vi "Get Data.vi"(8 "error in (no error)":errorcluster, 11 "Red Pitaya Digitizer in":refnum<class "Red Pitaya Digitizer.lvclass">) -> (0 "error out":errorcluster, 3 "Red Pitaya Digitizer out":refnum<class "Red Pitaya Digitizer.lvclass">)   [LabVIEW 2015, in "Red Pitaya Digitizer.lvclass"]
uses:
  Red Pitaya Digitizer.lvclass
  Red Pitaya Digitizer.lvclass/Red Pitaya Digitizer.ctl
  Read RP Instrument.lvclass.vi
  NHMFL_Core/Libraries/Red Pitaya/RP Core/RP Instrument/RP Instrument.lvclass
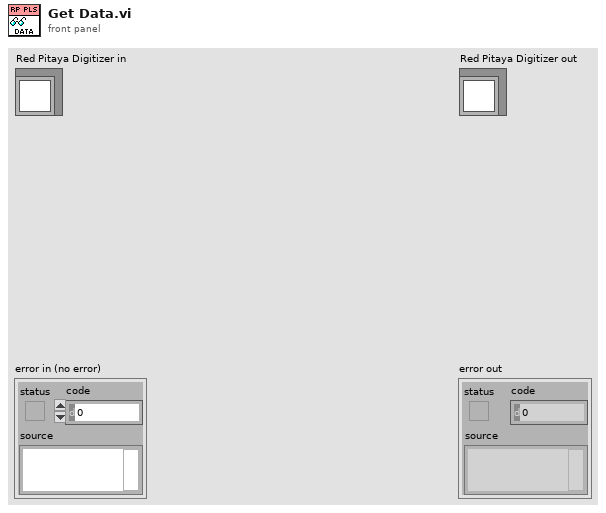
[diagram p1: front panel]
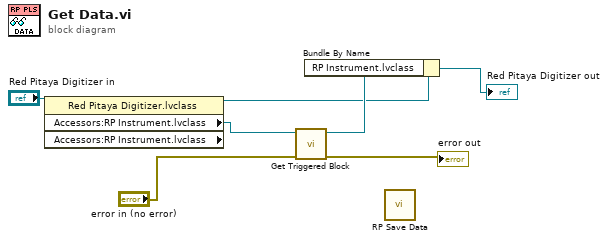
[diagram p0: block diagram]
diagram:
  n1 = property class="Red Pitaya Digitizer.lvclass" props=["Accessors:RP Instrument.lvclass", "Accessors:RP Instrument.lvclass"](reference="Red Pitaya Digitizer in") -> (reference out=w2:refnum<class "Red Pitaya Digitizer.lvclass">, "Accessors:RP Instrument.lvclass"=w1:refnum<class "RP Instrument.lvclass">)  [unwired: 1 in, 2 out]
  n2 = call-dynamic "Get Triggered Block.vi"("error in (no error)"="error in (no error)", "RP Instrument in"=w1) -> ("error out"=→"error out":errorcluster, "RP Instrument out"=w6:refnum<class "RP Instrument.lvclass">)  [unwired: 7 in, 1 out]
  n3 = Bundle By Name(cluster=w2, "RP Instrument.lvclass"=w6) -> (→"Red Pitaya Digitizer out":refnum<class "Red Pitaya Digitizer.lvclass">)
  n4 = call "RP Save Data.vi"() -> ()  [unwired: 8 in, 4 out]
